vi "Reset.vi"(8 "error in (no error)":errorcluster, 11 "VISA resource name":refnum<visa-resource-name>) -> (0 "error out":errorcluster, 3 "VISA resource name out":refnum<visa-resource-name>)   [LabVIEW 2020, in "EFD Ultimus V.lvlib"]
doc: "Resets the Ultimus V and then sends a set of default setup commands to the Ultimus V."
uses:
  EFD Ultimus V.lvlib
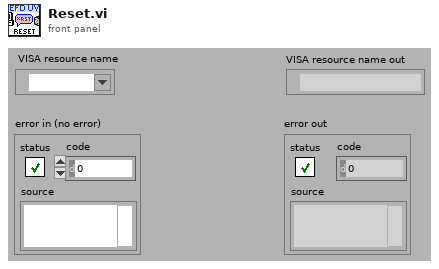
[diagram p1: front panel]
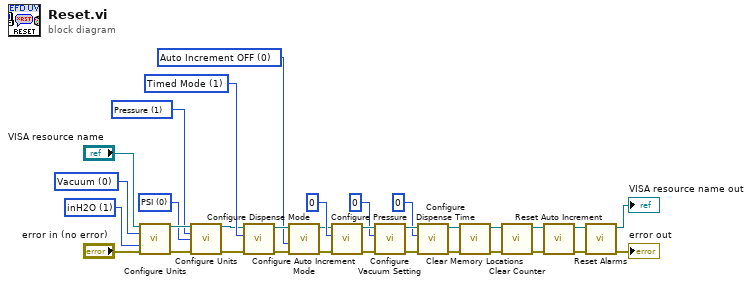
[diagram p0: block diagram]
diagram:
  w1 = u16 0 items=["Auto Increment OFF", "Timer Mode", "Counter Mode", "Auto Sequence Mode"] ("Auto Increment (Timer)")
  w6 = u16 0 items=["PSI", "BAR", "KPA"] ("Pressure Units (PSI/BAR/KPA)")
  w7 = u16 1 items=["Vacuum ", "Pressure"] ("Measurement Type (Pressure/Vacuum)")
  w12 = u16 1 items=["Steady Mode", "Timed Mode"] ("Ultimus V Mode (Timed/Steady)")
  w13 = u16 1 items=["KPA", "inH2O", "inHg", "mmHg", "TORR"] ("Vacuum Units (inH20,inHg,mmHg,KPA,TORR)")
  w14 = u16 0 items=["Vacuum ", "Pressure"] ("Measurement Type (Pressure/Vacuum)")
  n1 = call "Configure Units.vi"("VISA resource name"="VISA resource name", "Measurement Type (0: Vacuum)"=w14, "Vacuum Units (1: inH20)"=w13, "error in (no error)"="error in (no error)") -> ("VISA resource name out"=w11:refnum<visa-resource-name>, "error out"=w10:errorcluster)  [unwired: 10 in]
  n2 = call "Configure Units.vi"("VISA resource name"=w11, "Measurement Type (0: Vacuum)"=w7, "Pressure Units (0: PSI)"=w6, "error in (no error)"=w10) -> ("VISA resource name out"=w9:refnum<visa-resource-name>, "error out"=w8:errorcluster)  [unwired: 10 in]
  n3 = call "Configure Dispense Mode.vi"("error in (no error)"=w8, "Dispense Mode (0: Steady)"=w12, "VISA resource name"=w9) -> ("error out"=w4:errorcluster, "VISA resource name out"=w3:refnum<visa-resource-name>)  [unwired: 7 out]
  n4 = call "Configure Auto Increment Mode.vi"("error in (no error)"=w4, "Auto Increment (1:Timer)"=w1, "VISA resource name"=w3) -> ("error out"=w5:errorcluster, "VISA resource name out"=w2:refnum<visa-resource-name>)  [unwired: 7 in]
  n5 = call "Configure Pressure.vi"("error in (no error)"=w5, "Pressure Setting (0000)"=i64 0 ("Set Pressure (pppp)"), "VISA resource name"=w2) -> ("error out"=w22:errorcluster, "VISA resource name out"=w24:refnum<visa-resource-name>)  [unwired: 7 out]
  n6 = call "Configure Vacuum Setting.vi"("error in (no error)"=w22, "Vacuum Setting (0000)"=i64 0 ("Set Vacuum (vvvv)"), "VISA resource name"=w24) -> ("error out"=w23:errorcluster, "VISA resource name out"=w25:refnum<visa-resource-name>)  [unwired: 7 out]
  n7 = call "Configure Dispense Time.vi"("error in (no error)"=w23, "Dispense Time (0000)"=0 ("Set Time (ttttt)"), "VISA resource name"=w25) -> ("error out"=w33:errorcluster, "VISA resource name out"=w32:refnum<visa-resource-name>)  [unwired: 7 out]
  n8 = call "Clear Memory Locations.vi"("error in (no error)"=w33, "VISA resource name"=w32) -> ("error out"=w26:errorcluster, "VISA resource name out"=w29:refnum<visa-resource-name>)  [unwired: 8 out]
  n9 = call "Clear Counter.vi"("error in (no error)"=w26, "VISA resource name"=w29) -> ("error out"=w27:errorcluster, "VISA resource name out"=w30:refnum<visa-resource-name>)  [unwired: 8 out]
  n10 = call "Reset Auto Increment.vi"("error in (no error)"=w27, "VISA resource name"=w30) -> ("error out"=w28:errorcluster, "VISA resource name out"=w31:refnum<visa-resource-name>)  [unwired: 8 out]
  n11 = call "Reset Alarms.vi"("error in (no error)"=w28, "VISA resource name"=w31) -> ("error out"=→"error out":errorcluster, "VISA resource name out"=→"VISA resource name out":refnum<visa-resource-name>)  [unwired: 8 out]
